vi "Filtrado Digital.vi"() -> ()   [LabVIEW 2018]
uses:
  <vilib>/express/express analysis/Spectral/Block/exnSpectralBlock spectral measurements peak poly.vi
  <vilib>/express/express analysis/Spectral/Block/exnSpectralBlock spectral measurements peak DDT.vi
  <vilib>/express/express analysis/Spectral/XNode/ExpressSpectralMeasurementsBlockNode.xnode
  <vilib>/measure/NI_MABase.lvlib
panel:
  out "Filtered Signal":dynamicdata(graph)
  out "Waveform Graph":dynamicdata(graph)
  out "Grafica de Entrada":dynamicdata(graph)
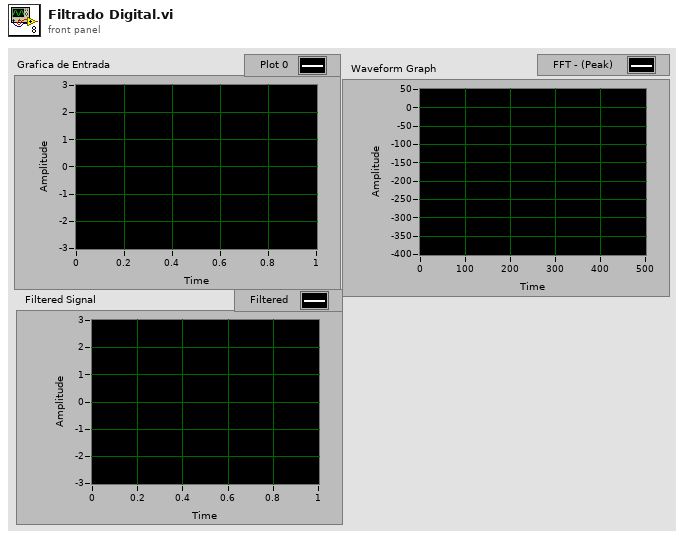
[diagram p1: front panel]
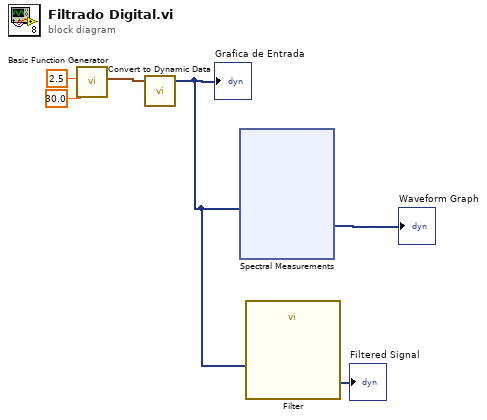
[diagram p0: block diagram]
diagram:
  n1 = call <vilib>:"Basic Function Generator.vi"("amplitude"=2.5, "frequency"=30.0) -> ("signal out"=w4:waveform(dbl))  [unwired: 7 in, 2 out]
  n2 = call "Convert to Dynamic Data"("Waveform"=w4) -> ("Dynamic Data Type"=w2:dynamicdata)  [unwired: 3 in]
  "Grafica de Entrada" <- w2
  n3 = xnode "Spectral Measurements"("Signals"=w2) -> ("FFT - (Peak)"=→"Waveform Graph":dynamicdata)  [unwired: 1 in, 2 out]
  n4 = call "Filter"("Signal"=w2) -> ("Filtered Signal"=→"Filtered Signal":dynamicdata)  [unwired: 9 in, 1 out]
